vi "NIFPGA-MCS.set bin width.vi"(0 "i ref in":refnum<vi>, 2 "binWidth [us]":dbl, 3 "ms timeout (10000)":i32=10000, 5 "error in (no error)":errorcluster) -> (14 "i ref out":refnum<vi>, 16 "binWidth out [us]":dbl, 17 "timed out":bool, 19 "error out":errorcluster)   [LabVIEW 2014, in "NIFPGA-MCS.lvlib"]
doc: "Sets the width of a bin in a spectrum of the MCS."
uses:
  NIFPGA-MCS.lvlib
  CSCore/CSApplicationBaseClasses/MCSBase/MCSBase.directionType.ctl
  CSCore/CSApplicationBaseClasses/MCSBase/MCSBase.serviceType.ctl
  CSlibraries/UtilityLib/UtilityLib.valueStatus.ctl
  CSinstr.lib/NI-FPGA-MCS/host/instrumentDriver/NI-FPGA-MCS_Driver.lvlib
  CSCore/CSApplicationBaseClasses/DeviceBase/DeviceBase.lvlib
  CSCore/CSApplicationBaseClasses/MCSBase/MCSBase.lvlib
  CSlibraries/UtilityLib/UtilityLib.lvlib
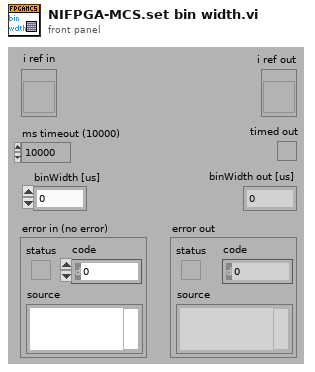
[diagram p1: front panel]
types:
  T1 = typedef "UtilityLib.lvlib/UtilityLib.valueStatus.ctl" = enum16{"no info available", "stand by/off", "on", "warning", "alarm/malfunction", "not implemented", "user action required", "important information", "system default", "control default", "indicator default", "button default"}
  T2 = typedef "MCSBase.lvlib/MCSBase.serviceType.ctl" = enum16{"counts", "totalCounts", "binWidth", "nOfBins", "nOfRecords", "status", "discrLevel", "discrSlope", "triggerLevel", "triggerSlope"}
  T3 = typedef "MCSBase.lvlib/MCSBase.directionType.ctl" = enum16{"unknown", "update actual value", "update nominal value", "update both"}
  T4 = typedef "NIFPGA-MCS.lvlib/NIFPGA-MCS.i attribute.ctl" = cluster{"fpgaViRef":T5}
  T5 = typedef "NI-FPGA-MCS_Driver.lvlib/fpga_vi_ref.ctl" = refnum<k20>
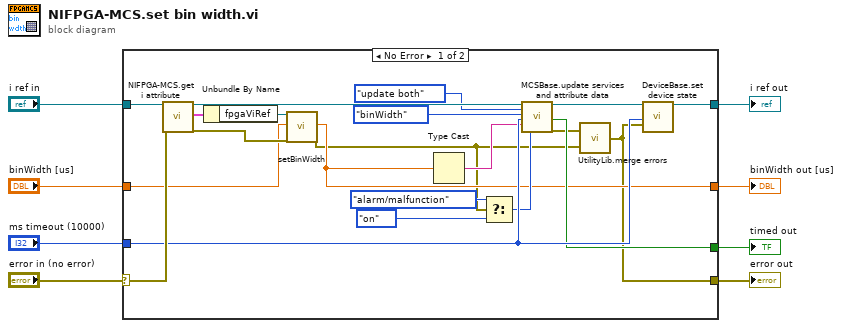
[diagram p0: block diagram]
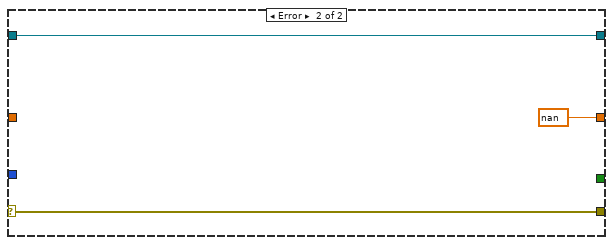
[diagram p2: hidden frame]
diagram:
  n1 = case shown="No Error" "error in (no error)" {
    selector: "error in (no error)" -> [w28 w31]
    tunnel: "i ref in" -> [w29 w32]
    tunnel: [w25 w32] -> w6
    tunnel: [w9 w31] -> w5
    tunnel: "ms timeout (10000)" -> [w21 _]
    tunnel: [w20 _] -> w3
    tunnel: "binWidth [us]" -> [w13 _]
    tunnel: [w12 nan ("binWidth [us] out")] -> w1
    frame No Error {
      n2 = call "NIFPGA-MCS.get i attribute.vi"("i ref in"=w29, "error in (no error)"=w28) -> ("i ref out"=w23:refnum<vi>, "i attribute"=w26:T4, "error out"=w27:errorcluster)  [unwired: 15 in]
      n3 = Unbundle By Name(w26) -> ("fpgaViRef"=w24:T5)
      n4 = call "setBinWidth.vi"("fpga_vi_ref"=w24, "binWidth [us]"=w13, "error in (no error)"=w27) -> ("binWidth [us] out"=w12:dbl, "error out"=w10:errorcluster)  [unwired: 14 in, 1 out]
      n5 = Type Cast(x=w12) -> (*(type *) &x=w17:string)  [unwired: 1 in]
      n6 = Select(t=UtilityLib.valueStatus."alarm/malfunction", s=w10, f=UtilityLib.valueStatus."on" ("quality")) -> (s? t:f=w14:T1)
      n7 = call "MCSBase.update services and attribute data.vi"("i ref in"=w23, "direction"=MCSBase.directionType."update both", "service"=MCSBase.serviceType."binWidth", "ms timeout (10000)"=w21, "value"=w17, "quality"=w14) -> ("i ref out"=w22:refnum<vi>, "timed out"=w20:bool, "error out"=w11:errorcluster)  [unwired: 11 in]
      n8 = call "UtilityLib.merge errors.vi"("error2 (no error)"=w10, "error1 (no error)"=w11) -> ("error out"=w9:errorcluster)
      n9 = call "DeviceBase.set device state.vi"("i ref in"=w22, "ms timeout (10000)"=w21, "device error"=w9) -> ("i ref out"=w25:refnum<vi>)  [unwired: 14 in, 2 out]
    }
    frame Error {
    }
  }
  "error out" <- w5
  "i ref out" <- w6
  "timed out" <- w3
  "binWidth out [us]" <- w1
